vi "MFC.vi"() -> ()   [LabVIEW 2013]
uses:
  Users/Administrator/Desktop/MKS modbus Driver Library V1_0 BETA RELEASE/MKS/Product/MFC/Type Definitions/Modbus Action.ctl
  GlobalStop.vi
panel:
  out "Numerisch 3":dbl
  out "Numerisch 2":dbl
  out "Numerisch":dbl
  out "error out 5":errorcluster
  out "error out 4":errorcluster
  out "error out 3":errorcluster
  out "error out 2":errorcluster
  out "error out":errorcluster
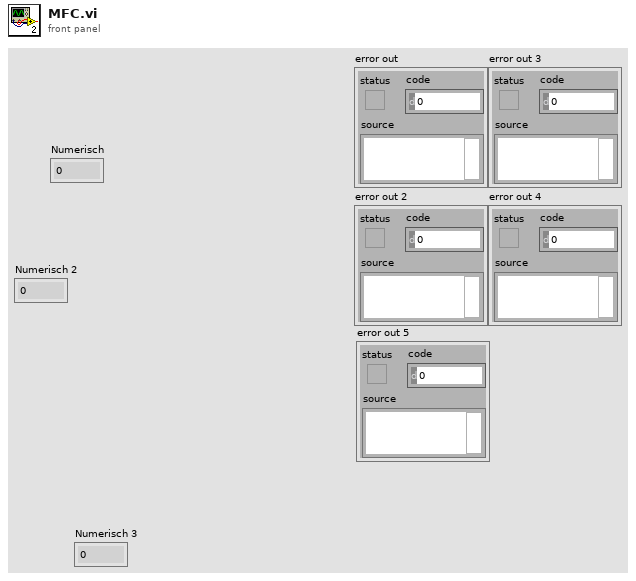
[diagram p1: front panel]
types:
  T1 = typedef "Modbus Action.ctl" = enum16{"Read", "Write"}
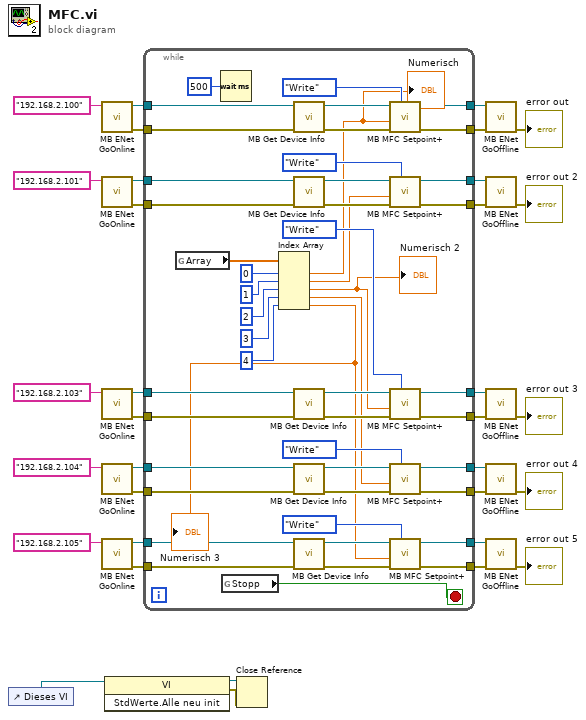
[diagram p0: block diagram]
diagram:
  n1 = control-ref of="Dieses VI"() -> (w3:refnum<vi>)
  n2 = call "MB ENet GoOnline.vi"("IP Address"="192.168.2.100") -> ("error out"=w11:errorcluster, "TCP Ref"=w26:refnum<k5>)  [unwired: 8 in, 1 out]
  n3 = call "MB ENet GoOnline.vi"("IP Address"="192.168.2.101") -> ("error out"=w28:errorcluster, "TCP Ref"=w22:refnum<k5>)  [unwired: 8 in, 1 out]
  n4 = call "MB ENet GoOnline.vi"("IP Address"="192.168.2.103") -> ("error out"=w27:errorcluster, "TCP Ref"=w23:refnum<k5>)  [unwired: 8 in, 1 out]
  n5 = call "MB ENet GoOnline.vi"("IP Address"="192.168.2.104") -> ("error out"=w9:errorcluster, "TCP Ref"=w25:refnum<k5>)  [unwired: 8 in, 1 out]
  n6 = call "MB ENet GoOnline.vi"("IP Address"="192.168.2.105") -> ("error out"=w10:errorcluster, "TCP Ref"=w24:refnum<k5>)  [unwired: 8 in, 1 out]
  n7 = invoke class="VI" method="StdWerte.Alle neu init"(reference=w3) -> (reference out=w2:refnum<vi>, error out=w1:errorcluster)  [unwired: 2 in, 1 out]
  n8 = while {
    tunnel: w28 -> [w66]
    tunnel: w27 -> [w65]
    tunnel: w26 -> [w64]
    tunnel: w25 -> [w63]
    tunnel: w24 -> [w62]
    tunnel: w23 -> [w61]
    tunnel: w22 -> [w60]
    tunnel: [w59] -> w21
    tunnel: [w58] -> w20
    tunnel: [w57] -> w19
    tunnel: [w56] -> w18
    tunnel: [w55] -> w17
    tunnel: [w54] -> w16
    tunnel: [w53] -> w15
    tunnel: [w52] -> w14
    tunnel: [w51] -> w13
    tunnel: [w50] -> w12
    tunnel: w11 -> [w49]
    tunnel: w10 -> [w48]
    tunnel: w9 -> [w47]
    stop <- w34 stop-if-true
    n9 = global read "GlobalMFC.vi" "Array"() -> (w46:dbl[])
    n10 = Wait (ms)(milliseconds to wait=u32 500 ("Zu wartende ms")) -> ()  [unwired: 1 out]
    n11 = global read "GlobalStop.vi" "Stopp"() -> (w34:bool)
    n12 = Index Array(array=w46, index #1=0 ("Index"), index #2=1 ("Index"), index #3=2 ("Index"), index #4=3 ("Index"), index #5=4 ("Index")) -> (element #1=w36:dbl, element #2=w45:dbl, element #3=w37:dbl, element #4=w44:dbl, element #5=w35:dbl)
    "Numerisch" <- w36
    "Numerisch 3" <- w35
    "Numerisch 2" <- w37
    n13 = call "MB Get Device Info.vi"("error in (no error)"=w49, "TCP Ref:ValBlock"=w64) -> ("error out"=w68:errorcluster, "dup TCP Ref:ValBlock"=w67:refnum<k5>)  [unwired: 7 in, 1 out]
    n14 = call "MB Get Device Info.vi"("error in (no error)"=w66, "TCP Ref:ValBlock"=w60) -> ("error out"=w76:errorcluster, "dup TCP Ref:ValBlock"=w75:refnum<k5>)  [unwired: 7 in, 1 out]
    n15 = call "MB Get Device Info.vi"("error in (no error)"=w65, "TCP Ref:ValBlock"=w61) -> ("error out"=w74:errorcluster, "dup TCP Ref:ValBlock"=w73:refnum<k5>)  [unwired: 7 in, 1 out]
    n16 = call "MB Get Device Info.vi"("error in (no error)"=w47, "TCP Ref:ValBlock"=w63) -> ("error out"=w70:errorcluster, "dup TCP Ref:ValBlock"=w69:refnum<k5>)  [unwired: 7 in, 1 out]
    n17 = call "MB Get Device Info.vi"("error in (no error)"=w48, "TCP Ref:ValBlock"=w62) -> ("error out"=w72:errorcluster, "dup TCP Ref:ValBlock"=w71:refnum<k5>)  [unwired: 7 in, 1 out]
    n18 = call "MB MFC Setpoint+.vi"("Action"=Modbus_Action."Write", "error in (no error)"=w68, "Setpoint"=w36, "TCP Ref"=w67) -> ("error out"=w51:errorcluster, "dup TCP Ref"=w50:refnum<k5>)  [unwired: 5 in, 1 out]
    n19 = call "MB MFC Setpoint+.vi"("Action"=Modbus_Action."Write", "error in (no error)"=w76, "Setpoint"=w45, "TCP Ref"=w75) -> ("error out"=w59:errorcluster, "dup TCP Ref"=w58:refnum<k5>)  [unwired: 5 in, 1 out]
    n20 = call "MB MFC Setpoint+.vi"("Action"=Modbus_Action."Write", "error in (no error)"=w74, "Setpoint"=w37, "TCP Ref"=w73) -> ("error out"=w57:errorcluster, "dup TCP Ref"=w56:refnum<k5>)  [unwired: 5 in, 1 out]
    n21 = call "MB MFC Setpoint+.vi"("Action"=Modbus_Action."Write", "error in (no error)"=w70, "Setpoint"=w44, "TCP Ref"=w69) -> ("error out"=w53:errorcluster, "dup TCP Ref"=w52:refnum<k5>)  [unwired: 5 in, 1 out]
    n22 = call "MB MFC Setpoint+.vi"("Action"=Modbus_Action."Write", "error in (no error)"=w72, "Setpoint"=w35, "TCP Ref"=w71) -> ("error out"=w55:errorcluster, "dup TCP Ref"=w54:refnum<k5>)  [unwired: 5 in, 1 out]
  }
  n23 = Close Reference(reference=w2, error in (no error)=w1) -> ()  [unwired: 1 out]
  n24 = call "MB ENet GoOffline.vi"("error in (no error)"=w13, "TCP Ref:ValBlock"=w12) -> ("error out"=→"error out":errorcluster)  [unwired: 7 in, 2 out]
  n25 = call "MB ENet GoOffline.vi"("error in (no error)"=w21, "TCP Ref:ValBlock"=w20) -> ("error out"=→"error out 2":errorcluster)  [unwired: 7 in, 2 out]
  n26 = call "MB ENet GoOffline.vi"("error in (no error)"=w19, "TCP Ref:ValBlock"=w18) -> ("error out"=→"error out 3":errorcluster)  [unwired: 7 in, 2 out]
  n27 = call "MB ENet GoOffline.vi"("error in (no error)"=w15, "TCP Ref:ValBlock"=w14) -> ("error out"=→"error out 4":errorcluster)  [unwired: 7 in, 2 out]
  n28 = call "MB ENet GoOffline.vi"("error in (no error)"=w17, "TCP Ref:ValBlock"=w16) -> ("error out"=→"error out 5":errorcluster)  [unwired: 7 in, 2 out]
